vi "SSL Detection Balls Delete Invalids.vi"(11 "Balls In":T1[](array[typedef])) -> (3 "Balls Out":T1[](array[typedef]))   [LabVIEW 2016]
uses:
  SSL Detection Ball.ctl
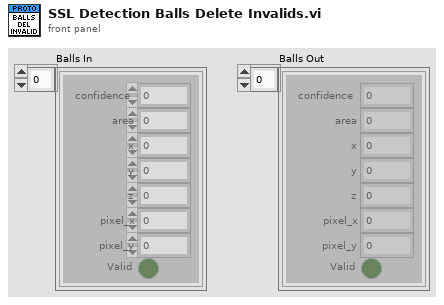
[diagram p1: front panel]
types:
  T1 = typedef "SSL Detection Ball.ctl" = cluster{"x":sgl, "area":u32, "confidence":sgl, "y":sgl, "z":sgl, "pixel_x":sgl, "pixel_y":sgl, "Valid":bool}
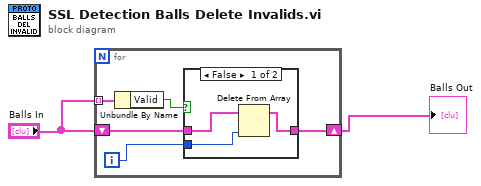
[diagram p0: block diagram]
diagram:
  n1 = for {
    tunnel: "Balls In" -> [w7] mode=indexing
    shift-right: [w3] -> w2
    shift-left: "Balls In" -> [w5]
    i -> [w4]
    n2 = Unbundle By Name(w7) -> ("Valid"=w6:bool)
    n3 = case shown="False" w6 {
      tunnel: w5 -> [w10 w11]
      tunnel: w4 -> [w9 _]
      tunnel: [w8 w11] -> w3
      frame False {
        n4 = Delete From Array(array=w10, index=w9) -> (array with subset deleted=w8:T1[])  [unwired: 1 in, 1 out]
      }
      frame True {
      }
    }
  }
  "Balls Out" <- w2
